vi "GetStripIndex.vi"(1 "Channel no array in":dbl[](array[numeric]) format="%.2f", 2 "Channel no. in":i32=1 min=0 max=769 step=1) -> (0 "Index out":i32)   [LabVIEW 2019]
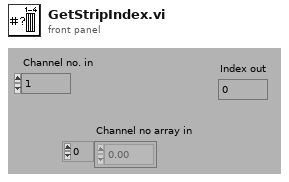
[diagram p1: front panel]
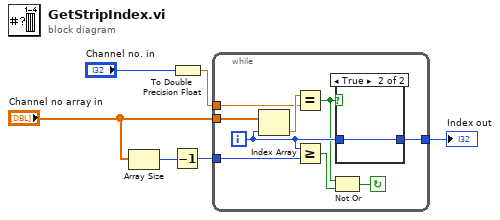
[diagram p0: block diagram]
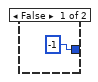
[diagram p2: hidden frame]
diagram:
  n1 = Array Size(array="Channel no array in") -> (size(s)=w2:i32)
  n2 = Decrement(x=w2) -> (x-1=w1:i32)
  n3 = To Double Precision Float(number="Channel no. in") -> (double precision float=w5:dbl)
  n4 = while {
    tunnel: "Channel no array in" -> [w15]
    tunnel: w5 -> [w13]
    tunnel: [w12] -> w4
    tunnel: w1 -> [w11]
    i -> [w10]
    stop <- w7 continue-if-true
    n5 = Index Array(array=w15, index=w10) -> (element=w14:dbl)
    n6 = Equal?(x=w14, y=w13) -> (x = y?=w9:bool)
    n7 = Greater Or Equal?(x=w10, y=w11) -> (x >= y?=w8:bool)
    n8 = Not Or(1:w8, 2:w9) -> (0:w7:bool)
    n9 = case shown="True" w9 {
      tunnel: w10 -> [_ w17]
      tunnel: [-1 w17] -> w12
      frame False {
      }
      frame True {
      }
    }
  }
  "Index out" <- w4
